vi "Scripting_ConvertBaseClassToSubClass_UpdateNativeCreate.vi"(7 "AppRef":refnum<vi>, 8 "error in (no error)":errorcluster, 9 "NewBaseClassInitViPath":path=path "C:/Projects/P1G/N1_class/N1_Init.vi", 11 "CurrentBaseInitVI":path=path "C:/Projects/P1G/N2_class/N2_Init.vi") -> (0 "error out":errorcluster)   [LabVIEW 2014]
doc: "Use this template to build a VI to use as a subVI."
uses:
  <vilib>/Utility/miscctls.llb/LVPositionTypeDef.ctl
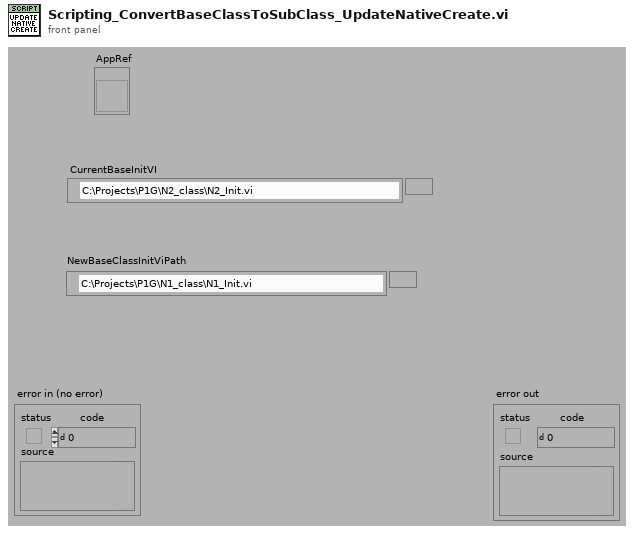
[diagram p1: front panel]
types:
  T1 = typedef "LVPositionTypeDef.ctl" = cluster{"Left":i32, "Top":i32}
  T2 = typedef "LVRectTypeDef.ctl" = cluster{"Left":i16, "Top":i16, "Right":i16, "Bottom":i16}
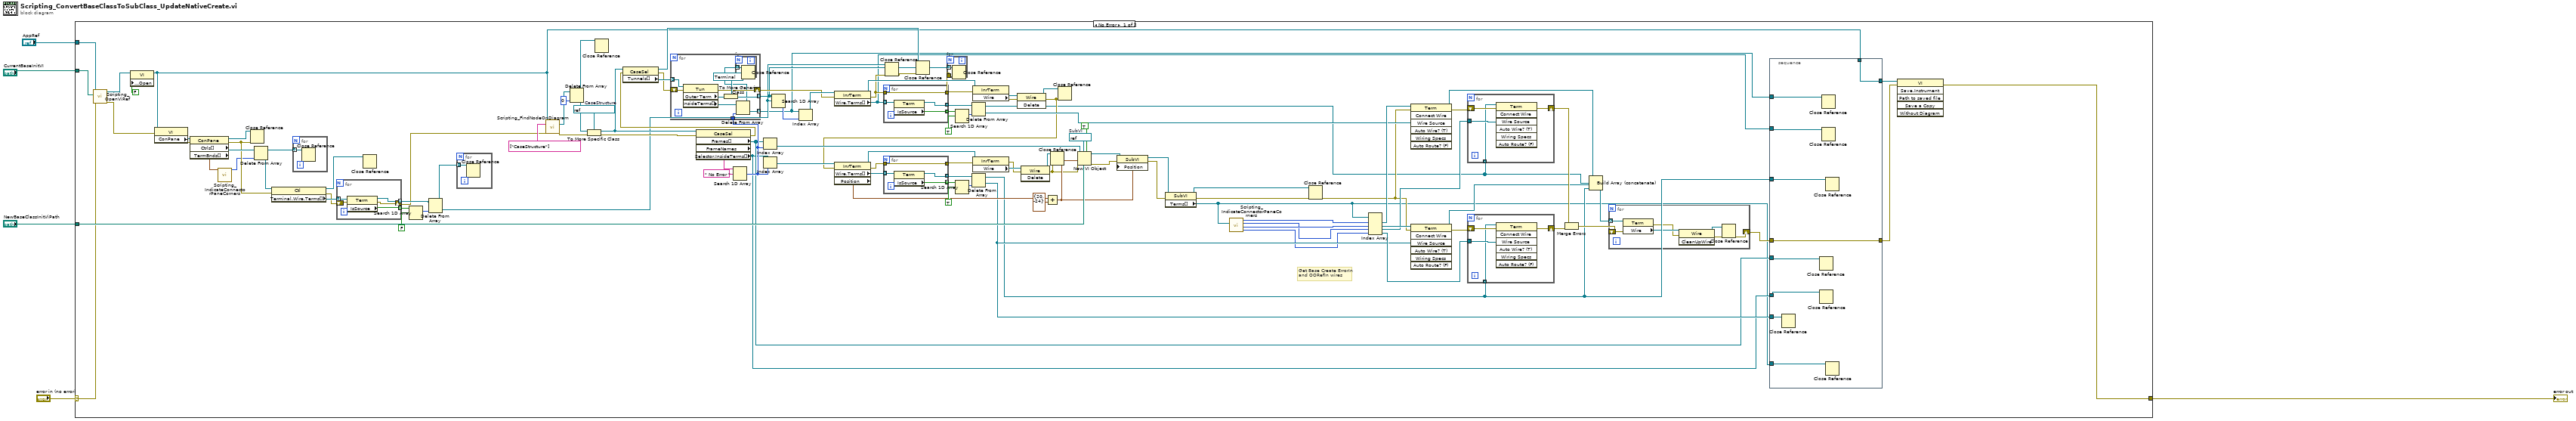
[diagram p0: block diagram]
diagram:
  n1 = case shown="No Error" "error in (no error)" {
    selector: "error in (no error)" -> [w100 w171]
    tunnel: [w24 w171] -> w4
    tunnel: "CurrentBaseInitVI" -> [w101 _]
    tunnel: "NewBaseClassInitViPath" -> [w119 _]
    tunnel: "AppRef" -> [w6 _]
    frame No Error {
      w111 = refnum<vi> refnum  # CaseStructure
      w118 = refnum<vi> refnum  # SubVI
      # "Get Base Create ErrorIn\nand OORefIn wires"
      n2 = call <resource>:"Scripting_OpenViRef.vi"("error in"=w100, "ViPath/ViName/Viref"=w101, "AppRef"=w6) -> ("error out"=w72:errorcluster, "vi reference"=w48:refnum<vi>)  [unwired: 6 in, 1 out]
      n3 = property class="VI"(reference=w48, "Front Panel.Open"=FALSE ("Front Panel Window:Open")) -> (reference out=w27:refnum<vi>)  [unwired: 1 in, 1 out]
      n4 = property class="VI"(reference=w27, error in=w72) -> (error out=w82:errorcluster, "ConPane"=w83:refnum<vi>)  [unwired: 1 out]
      n5 = property class="ConPane"(reference=w83, error in=w82) -> (reference out=w46:refnum<vi>, error out=w47:errorcluster, "Ctrls[]"=w81:refnum<vi>[], "TermBnds[]"=w9:T2[])
      n6 = call <resource>:"Scripting_IndicateConnectorPaneCorners.vi"("TermBnds[]"=w9) -> ("LeftTop"=w8:i32)  [unwired: 7 in, 3 out]
      n7 = Close Reference(reference=w46, error in (no error)=w47) -> ()  [unwired: 1 out]
      n8 = Delete From Array(array=w81, index=w8) -> (deleted portion=w79:refnum<vi>, array with subset deleted=w80:refnum<vi>[])  [unwired: 1 in]
      n9 = property class="Ctl"(reference=w79, error in=w47) -> (reference out=w45:refnum<vi>, error out=w73:errorcluster, "Terminal.Wire.Terms[]"=w74:refnum<vi>[])
      n10 = for {
        tunnel: w80 -> [w153] mode=indexing
        n11 = Close Reference(reference=w153) -> ()  [unwired: 1 in, 1 out]
      }
      n12 = for {
        tunnel: w74 -> [w152] mode=indexing
        tunnel: [w151] -> w78 mode=indexing
        tunnel: [w150] -> w75 mode=indexing
        shift-right: [w148] -> w68
        shift-left: w73 -> [w149]
        n13 = property class="Term"(reference=w152, error in=w149) -> (reference out=w150:refnum<vi>, error out=w148:errorcluster, "IsSource"=w151:bool)
      }
      n14 = Close Reference(reference=w45) -> ()  [unwired: 1 in, 1 out]
      n15 = Search 1D Array(1D array=w78, element=FALSE) -> (index of element=w76:i32)  [unwired: 1 in]
      n16 = Delete From Array(array=w75, index=w76) -> (deleted portion=w43:refnum<vi>, array with subset deleted=w71:refnum<vi>[])  [unwired: 1 in]
      n17 = for {
        tunnel: [w147] -> _ mode=indexing
        tunnel: w71 -> [w147] mode=indexing
        n18 = Close Reference(reference=w147) -> ()  [unwired: 1 in, 1 out]
      }
      n19 = call <resource>:"Scripting_FindNodeOnDiagram.vi"("ViRef(Ignored If Not Wired)"=w27, "NodeTypesToSearchFor"=string[] ["CaseStructure"], "error in (no error)"=w68) -> ("Nodes"=w42:refnum<vi>[], "error out"=w110:errorcluster)  [unwired: 15 in]
      n20 = Delete From Array(array=w42, index=0) -> (deleted portion=w41:refnum<vi>, array with subset deleted=w7:refnum<vi>[])  [unwired: 1 in]
      n21 = To More Specific Class(target class=w111, reference=w41, error in=w110) -> (specific class reference=w70:refnum<vi>, error out=w51:errorcluster)
      n22 = Close Reference(reference=w7) -> ()  [unwired: 1 in, 1 out]
      n23 = property class="CaseSel"(reference=w70, error in=w51) -> (error out=w50:errorcluster, "Frames[]"=w33:refnum<vi>[], "FrameNames"=w109:string[], "Selector.InsideTerms[]"=w32:refnum<vi>[])  [unwired: 1 out]
      n24 = property class="CaseSel"(reference=w70, error in=w50) -> (reference out=w38:refnum<vi>, error out=w53:errorcluster, "Tunnels[]"=w69:refnum<vi>[])
      n25 = Search 1D Array(1D array=w109, element=" No Error ") -> (index of element=w62:i32)  [unwired: 1 in]
      n26 = for {
        tunnel: w69 -> [w145] mode=indexing
        tunnel: [w142] -> w36 mode=indexing
        tunnel: w62 -> [w138]
        tunnel: [w137] -> w35 mode=indexing
        shift-right: [w140] -> w52
        shift-left: w53 -> [w141]
        n27 = property class="Tun"(reference=w145, error in=w141) -> (error out=w140:errorcluster, "Outer Term"=w144:refnum<vi>, "InsideTerms[]"=w139:refnum<vi>[])  [unwired: 1 out]
        n28 = To More Generic Class(target class=refnum<vi> refnum ("element"), reference=w144) -> (generic class reference=w142:refnum<vi>)
        n29 = Delete From Array(array=w139, index=w138) -> (deleted portion=w137:refnum<vi>, array with subset deleted=w136:refnum<vi>[])  [unwired: 1 in]
        n30 = for {
          tunnel: w136 -> [w146] mode=indexing
          n31 = Close Reference(reference=w146) -> ()  [unwired: 1 in, 1 out]
        }
      }
      n32 = Index Array(array=w33, index=w62) -> (element=w94:refnum<vi>)
      n33 = Index Array(array=w32, index=w62) -> (element=w107:refnum<vi>)
      n34 = Search 1D Array(1D array=w36, element=w43) -> (index of element=w61:i32)  [unwired: 1 in]
      n35 = Index Array(array=w35, index=w61) -> (element=w60:refnum<vi>)
      n36 = property class="InrTerm"(reference=w60, error in=w52) -> (reference out=w67:refnum<vi>, error out=w44:errorcluster, "Wire.Terms[]"=w34:refnum<vi>[])
      n37 = for {
        tunnel: w34 -> [w135] mode=indexing
        tunnel: [w134] -> w63 mode=indexing
        tunnel: [w133] -> w66 mode=indexing
        tunnel: [w132] -> w37
        tunnel: w44 -> [w132]
        n38 = property class="Term"(reference=w135) -> (reference out=w133:refnum<vi>, "IsSource"=w134:bool)  [unwired: 1 in, 1 out]
      }
      n39 = Close Reference(reference=w43, error in (no error)=w44) -> (error out=w39:errorcluster)
      n40 = Close Reference(reference=w38, error in (no error)=w39) -> ()  [unwired: 1 out]
      n41 = for {
        tunnel: w37 -> [_]
        tunnel: w36 -> [w127] mode=indexing
        n42 = Close Reference(reference=w127) -> ()  [unwired: 1 in, 1 out]
      }
      n43 = Search 1D Array(1D array=w63, element=TRUE) -> (index of element=w65:i32)  [unwired: 1 in]
      n44 = Delete From Array(array=w66, index=w65) -> (deleted portion=w55:refnum<vi>, array with subset deleted=w18:refnum<vi>[])  [unwired: 1 in]
      n45 = property class="InrTerm"(reference=w67, error in=w37) -> (error out=w58:errorcluster, "Wire"=w59:refnum<vi>)  [unwired: 1 out]
      n46 = invoke class="Wire" method="Delete"(reference=w59, error in=w58) -> (reference out=w30:refnum<vi>, error out=w31:errorcluster)  [unwired: 1 in, 1 out]
      n47 = property class="InrTerm"(reference=w107, error in=w31) -> (reference out=w97:refnum<vi>, error out=w99:errorcluster, "Wire.Terms[]"=w106:refnum<vi>[], "Position"=w93:T1)
      n48 = for {
        tunnel: w106 -> [w161] mode=indexing
        tunnel: [w160] -> w105 mode=indexing
        tunnel: [w159] -> w102 mode=indexing
        tunnel: [w158] -> w98
        tunnel: w99 -> [w158]
        n49 = property class="Term"(reference=w161) -> (reference out=w159:refnum<vi>, "IsSource"=w160:bool)  [unwired: 1 in, 1 out]
      }
      n50 = Search 1D Array(1D array=w105, element=TRUE) -> (index of element=w103:i32)  [unwired: 1 in]
      n51 = Delete From Array(array=w102, index=w103) -> (deleted portion=w84:refnum<vi>, array with subset deleted=w16:refnum<vi>[])  [unwired: 1 in]
      n52 = property class="InrTerm"(reference=w97, error in=w98) -> (error out=w95:errorcluster, "Wire"=w96:refnum<vi>)  [unwired: 1 out]
      n53 = invoke class="Wire" method="Delete"(reference=w96, error in=w95) -> (reference out=w28:refnum<vi>, error out=w29:errorcluster)  [unwired: 1 in, 1 out]
      n54 = Add(x=w93, y=T1 {"Left"=20, "Top"=-24}) -> (x+y=w89:T1)
      n55 = Close Reference(reference=w28, error in (no error)=w29) -> ()  [unwired: 1 out]
      n56 = Close Reference(reference=w30, error in (no error)=w31) -> ()  [unwired: 1 out]
      n57 = New VI Object(vi object class=w118, auto wire? (F)=TRUE, owner refnum=w94, position/next to=w89, 6:w119, 8:w29) -> (object refnum=w90:refnum<vi>, 0:w91:errorcluster)  [unwired: 2 in]
      n58 = property class="SubVI"(reference=w90, error in=w91, "Position"=w89) -> (reference out=w87:refnum<vi>, error out=w88:errorcluster)
      n59 = property class="SubVI"(reference=w87, error in=w88) -> (reference out=w114:refnum<vi>, error out=w115:errorcluster, "Terms[]"=w10:refnum<vi>[])
      n60 = call <resource>:"Scripting_IndicateConnectorPaneCorners.vi"("Terminals[]"=w10) -> ("RightLower"=w11:i32, "LeftLower"=w13:i32, "RightTop"=w12:i32, "LeftTop"=w14:i32)  [unwired: 7 in]
      n61 = Close Reference(reference=w114, error in (no error)=w115) -> (error out=w49:errorcluster)
      n62 = Index Array(array=w10, index #1=w14, index #2=w13, index #3=w12, index #4=w11) -> (element #1=w56:refnum<vi>, element #2=w116:refnum<vi>, element #3=w54:refnum<vi>, element #4=w85:refnum<vi>)
      n63 = invoke class="Term" method="Connect Wire"(reference=w56, error in=w49, "Wire Source"=w55) -> (reference out=w19:refnum<vi>, error out=w57:errorcluster)  [unwired: 4 in, 5 out]
      n64 = invoke class="Term" method="Connect Wire"(reference=w116, error in=w49, "Wire Source"=w84) -> (reference out=w17:refnum<vi>, error out=w86:errorcluster)  [unwired: 4 in, 5 out]
      n65 = for {
        shift-right: [w128] -> w22
        shift-left: w57 -> [w131]
        tunnel: w54 -> [w130]
        tunnel: w18 -> [w129] mode=indexing
        n66 = invoke class="Term" method="Connect Wire"(reference=w129, error in=w131, "Wire Source"=w130) -> (error out=w128:errorcluster)  [unwired: 4 in, 6 out]
      }
      n67 = for {
        shift-right: [w154] -> w23
        shift-left: w86 -> [w157]
        tunnel: w85 -> [w156]
        tunnel: w16 -> [w155] mode=indexing
        n68 = invoke class="Term" method="Connect Wire"(reference=w155, error in=w157, "Wire Source"=w156) -> (error out=w154:errorcluster)  [unwired: 4 in, 6 out]
      }
      n69 = Merge Errors(w22, w23) -> (w21:errorcluster)
      n70 = Build Array (concatenate)(w19, w18, w17, w16) -> (w15:refnum<vi>[])
      n71 = for {
        shift-right: [w121] -> w20
        shift-left: w21 -> [w122]
        tunnel: w15 -> [w120] mode=indexing
        n72 = property class="Term"(reference=w120, error in=w122) -> (error out=w125:errorcluster, "Wire"=w126:refnum<vi>)  [unwired: 1 out]
        n73 = invoke class="Wire" method="CleanUpWire"(reference=w126, error in=w125) -> (reference out=w123:refnum<vi>, error out=w124:errorcluster)  [unwired: 1 in, 1 out]
        n74 = Close Reference(reference=w123, error in (no error)=w124) -> (error out=w121:errorcluster)
      }
      n75 = stacked-sequence {
        tunnel: w10 -> [w162]
        tunnel: w16 -> [w165]
        tunnel: w84 -> [w170]
        tunnel: w20 -> [w168]
        tunnel: w35 -> [w167]
        tunnel: w34 -> [w166]
        tunnel: w33 -> [w164]
        tunnel: w32 -> [w163]
        tunnel: w27 -> [w169]
        tunnel: [w169] -> w26
        tunnel: [w168] -> w25
        frame #0 {
          n76 = Close Reference(reference=w170) -> ()  [unwired: 1 in, 1 out]
          n77 = Close Reference(reference=w164) -> ()  [unwired: 1 in, 1 out]
          n78 = Close Reference(reference=w163) -> ()  [unwired: 1 in, 1 out]
          n79 = Close Reference(reference=w166) -> ()  [unwired: 1 in, 1 out]
          n80 = Close Reference(reference=w167) -> ()  [unwired: 1 in, 1 out]
          n81 = Close Reference(reference=w165) -> ()  [unwired: 1 in, 1 out]
          n82 = Close Reference(reference=w162) -> ()  [unwired: 1 in, 1 out]
        }
      }
      n83 = invoke class="VI" method="Save.Instrument"(reference=w26, error in=w25) -> (error out=w24:errorcluster)  [unwired: 4 in, 5 out]
    }
    frame Error {
    }
  }
  "error out" <- w4
